vi "ATS_Trunc.vi"(6 "TruncValue":u32=4, 7 "Value":u32) -> (3 "NewValue":u32)   [LabVIEW 2010]
doc: "Truncate the input value to the lower nearest TruncValue.\n\nNewValue= Trunc(Value/TruncValue) * TruncValue"
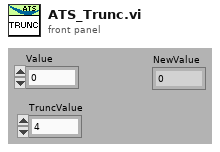
[diagram p1: front panel]
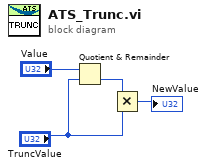
[diagram p0: block diagram]
diagram:
  n1 = Quotient & Remainder(x="Value", y="TruncValue") -> (floor(x/y)=w3:u32)  [unwired: 1 out]
  n2 = Multiply(x=w3, y="TruncValue") -> (x*y=→"NewValue":u32)
